vi "lab 2- 5.vi"() -> ()   [LabVIEW 2020]
panel:
  out "Boolean 4":bool
  out "Boolean 3":bool
  in  "Boolean 2":bool
  in  "Boolean":bool
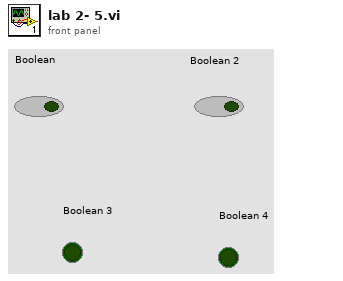
[diagram p1: front panel]
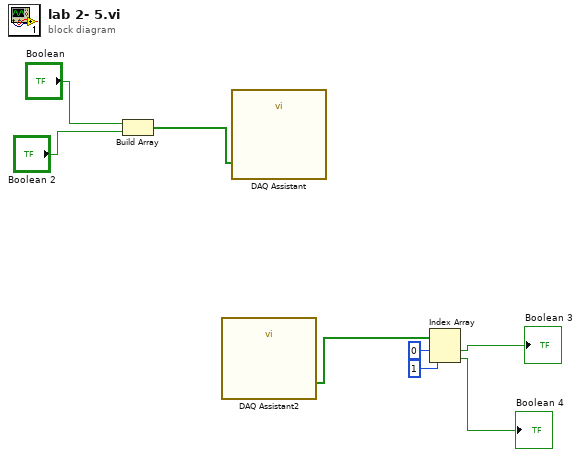
[diagram p0: block diagram]
diagram:
  n1 = Build Array("Boolean", "Boolean 2") -> (w6:bool[])
  n2 = call "DAQ Assistant2"() -> ("data"=w5:bool[])  [unwired: 17 in, 2 out]
  n3 = call "DAQ Assistant"("data"=w6) -> ()  [unwired: 17 in, 2 out]
  n4 = Index Array(array=w5, index #1=0 ("index"), index #2=1 ("index")) -> (element #1=→"Boolean 3":bool, element #2=→"Boolean 4":bool)
